vi "Read Status Code.vi"(8 "error in (no error)":errorcluster, 11 "response in":refnum<class "response.lvclass">) -> (0 "error out":errorcluster, 2 "status code":u16, 3 "response out":refnum<class "response.lvclass">)   [LabVIEW 2020, in "http.lvlib" / "response.lvclass"]
uses:
  response.lvclass
  response.lvclass/response.ctl
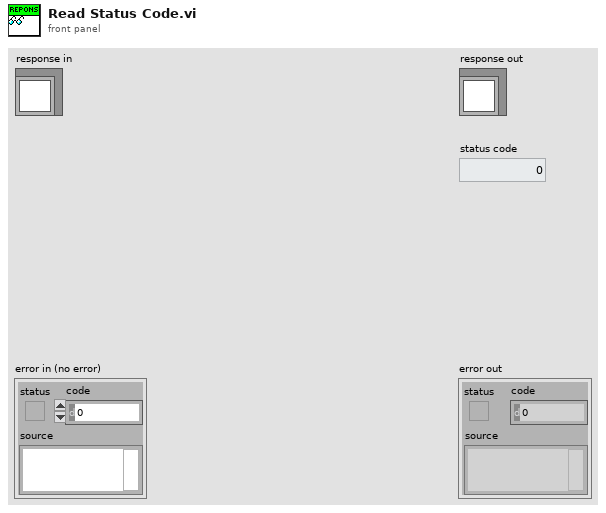
[diagram p1: front panel]
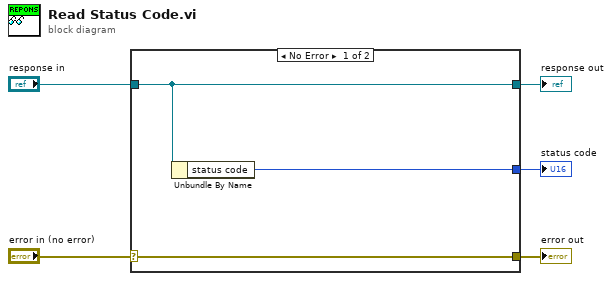
[diagram p0: block diagram]
diagram:
  n1 = case shown="No Error" "error in (no error)" {
    selector: "error in (no error)" -> [w8 w9]
    tunnel: [w8 w9] -> w4
    tunnel: [w7 w10] -> w2
    tunnel: "response in" -> [w7 w10]
    tunnel: [w6 _] -> w1
    frame No Error {
      n2 = Unbundle By Name(w7) -> ("status code"=w6:u16)
    }
    frame Error {
    }
  }
  "error out" <- w4
  "response out" <- w2
  "status code" <- w1
